vi "Unflatten UIP Value.vi"(10 "String Value":string, 11 "UIP In":refnum<class "DescriptionUIP.lvclass">) -> (0 "Error Out":errorcluster, 3 "UIP Out":refnum<class "DescriptionUIP.lvclass">)   [LabVIEW 2020, in "UIM.lvlib" / "DescriptionUIP.lvclass"]
uses:
  DescriptionUIP.lvclass
  DescriptionUIP.lvclass/DescriptionUIP.ctl
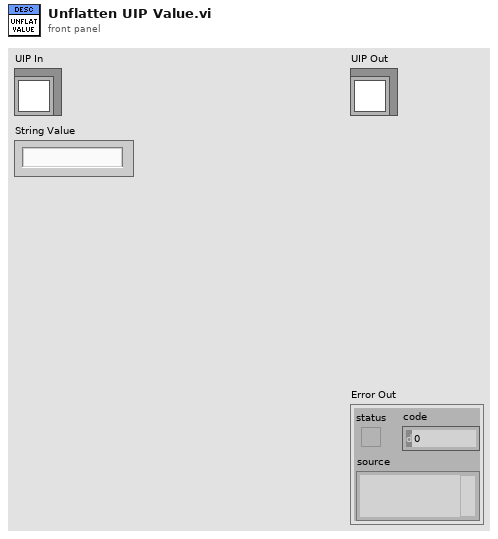
[diagram p1: front panel]
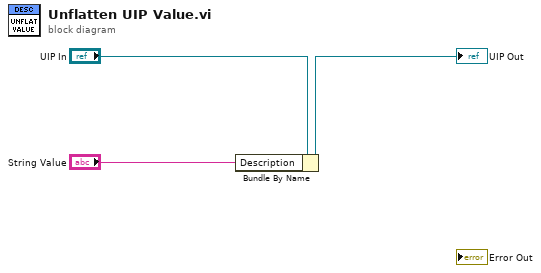
[diagram p0: block diagram]
diagram:
  n1 = Bundle By Name(cluster="UIP In", "Description"="String Value") -> (→"UIP Out":refnum<class "DescriptionUIP.lvclass">)
